vi "Serial_Auslesen_CO2Konzentration.vi"() -> ()   [LabVIEW 2023]
uses:
  aadfed2e-1559-dc4c-aa5c-28296088e4ea.vi
  <vilib>/Utility/file.llb/Write Delimited Spreadsheet (DBL).vi
  <vilib>/ptbypt/NI_PtbyPt.lvlib
panel:
  out "Mean CO2 Konzentration":dbl(graph)
  in  "Ref CO2":bool
  in  "Transmission Ref*1000:":i32
  in  "Verstärkung CO2:":i32
  in  "Verstärkung Ref:":i32
  out "CO2 Konzentration":dbl(graph)
  in  "Faktor Ch(CO2)*1000:":i32
  in  "Faktor CH(Referenz)*1000:":i32
  in  "Faktor k*1000:":i32
  in  "Abstand in cm:":i32
  in  "Absorbtionskoeffizient(CO2)*1000:":i32
  out "Mean Ref":dbl(graph)
  in  "Boolean":bool caption="In V aufnehmen"
  out "Mean A[V]:":dbl
  out "Aufnahme":dbl[](graph)
  in  "Aufnahme":bool
  in  "File":path
  in  "Transmit":bool
  in  "Sensor:":i8(knob) scale=1.0..4.0
  out "akt. Amplitude[V]:":dbl
  out "Mean Sig":dbl(graph)
  out "Ref":dbl(graph)
  in  "?":bool
  out "Waveform Chart":dbl(graph)
  in  "IR-Platine:":refnum<visa-resource-name>
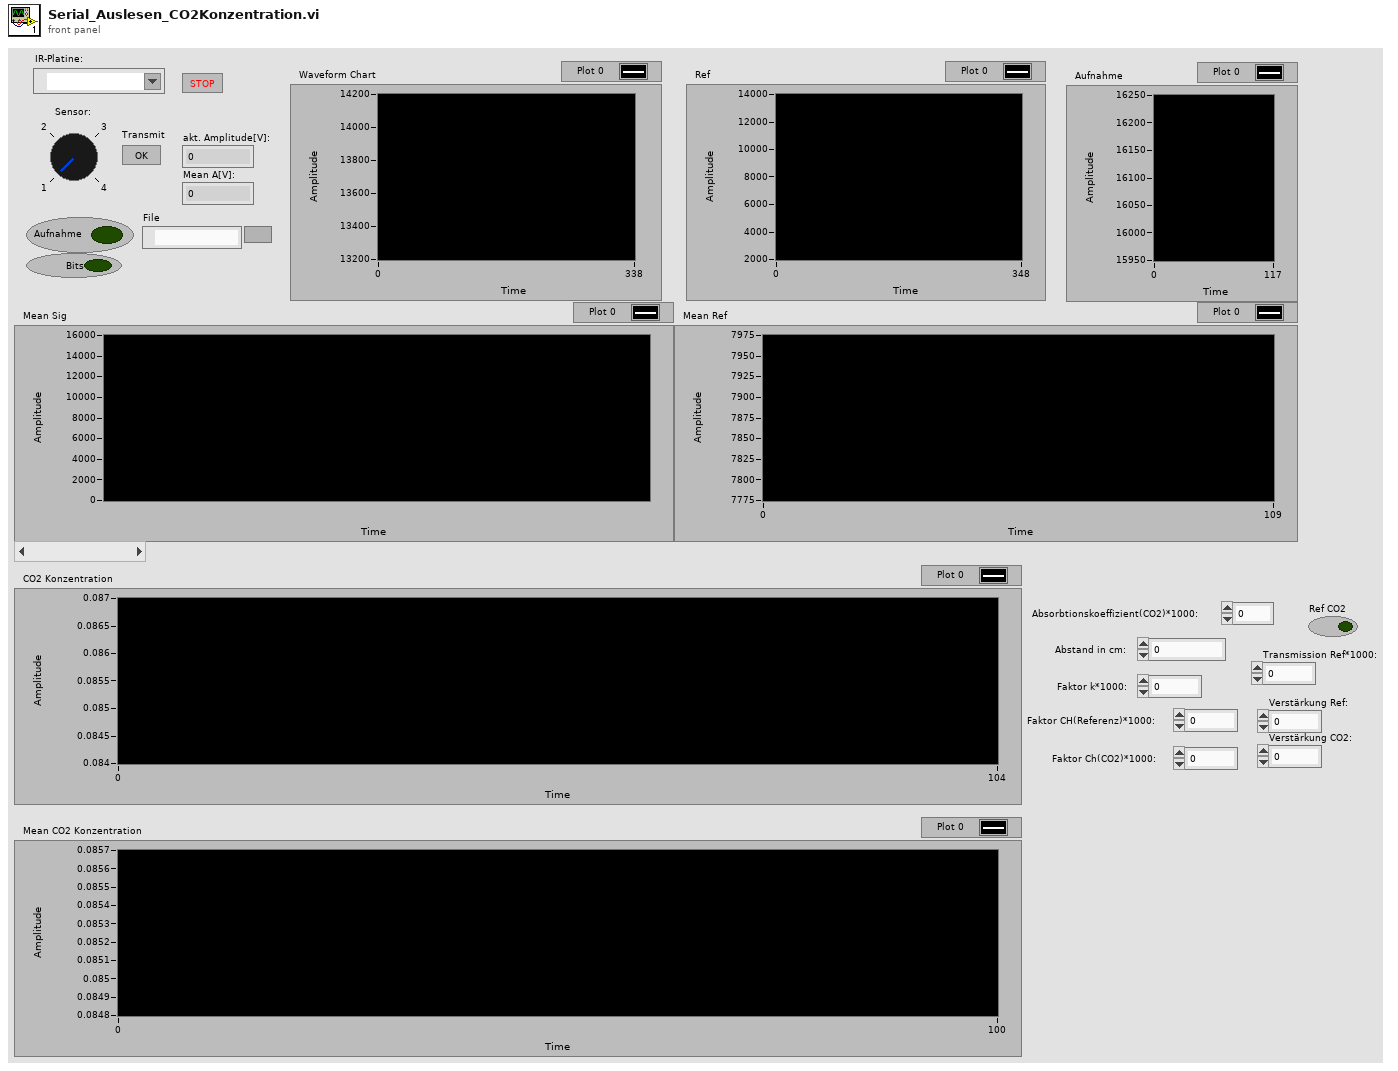
[diagram p1: front panel]
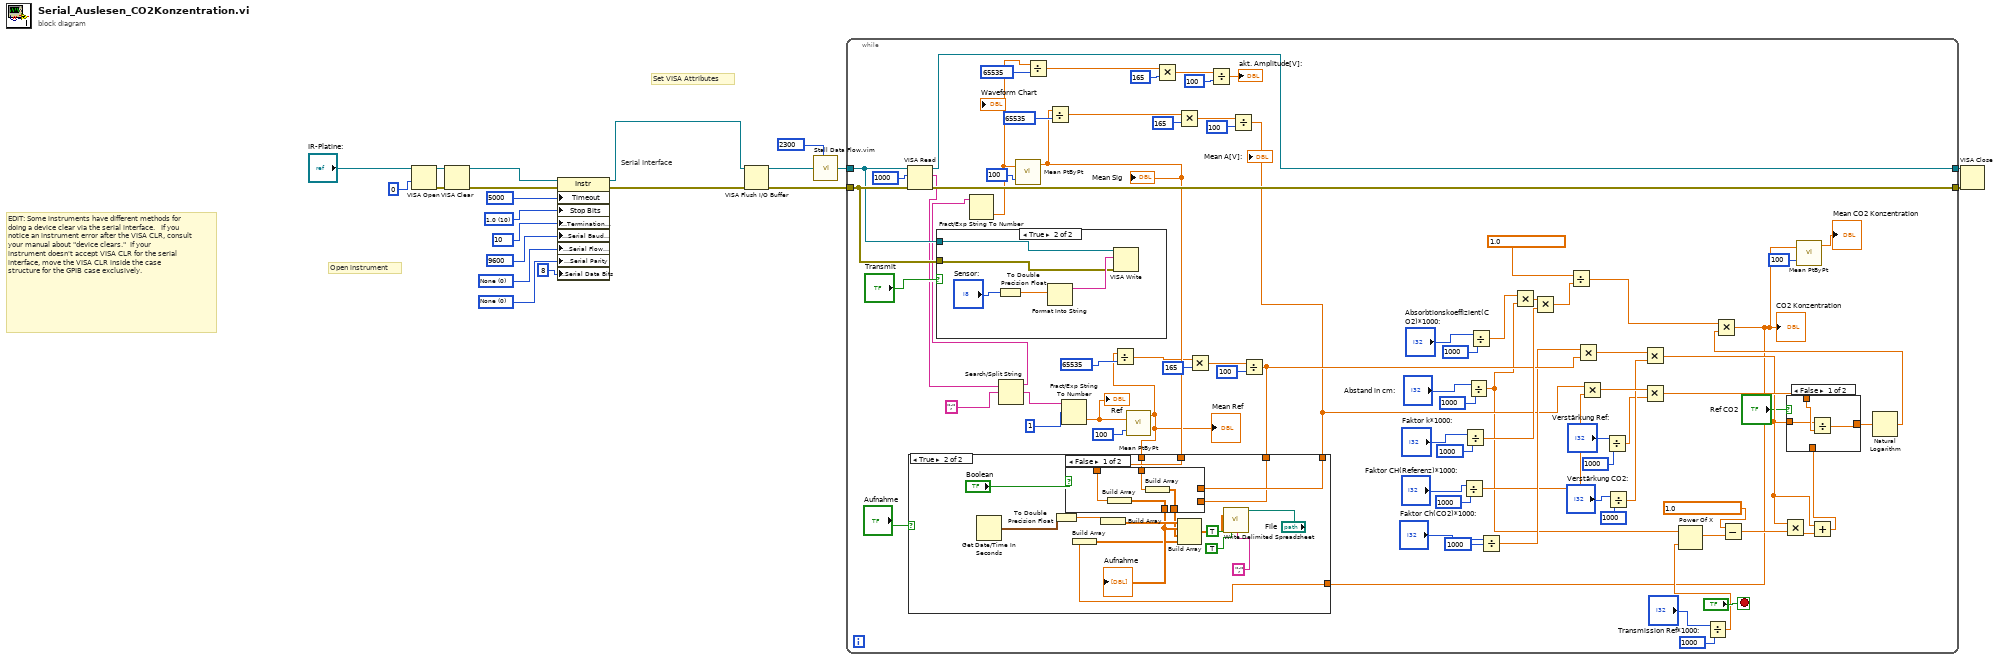
[diagram p0: block diagram]
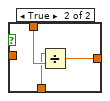
[diagram p2: hidden frame]
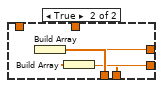
[diagram p4: hidden frame]
diagram:
  w9 = u16 0 items=["None", "Odd", "Even", "Mark", "Space"] ("Serial Settings:Parity")
  w10 = u16 0 items=["None", "XON/XOFF", "RTS/CTS", "XON/XOFF & RTS/CTS", "DTR/DSR", "XON/XOFF & DTR/DSR"] ("Serial Settings:Flow Control")
  w13 = u16 10 items=["1.0"=10, "1.5"=15, "2.0"=20] ("Serial Settings:Stop Bits")
  # "Serial Interface"
  # "EDIT: Some instruments have different methods for doing a device clear via the serial interface.   If you notice an instrument error after the VISA CLR, consult your manual about \"device clears.\"  If your instrument doesn't accept VISA CLR for the serial interface, move the VISA CLR inside the case  structure for the GPIB case exclusively."
  # "Set VISA Attributes"
  # "Open instrument"
  n1 = VISA Open(access mode=u32 0, VISA resource name="IR-Platine:") -> (VISA resource name=w19:refnum<visa-resource-name>, error out=w18:errorcluster)  [unwired: 3 in]
  n2 = VISA Clear(VISA resource name=w19, error in (no error)=w18) -> (VISA resource name out=w15:refnum<visa-resource-name>, error out=w1:errorcluster)
  n3 = property class="Instr"(reference=w15, error in=w1, "Timeout"=u32 5000 ("General Settings:Timeout Value"), "Stop Bits"=w13, "Message Based Settings:Termination Character"=u8 10, "Serial Settings:Serial Baud Rate"=u32 9600 ("Serial Settings:Baud Rate"), "Serial Settings:Serial Flow Control"=w10, "Serial Settings:Serial Parity"=w9, "Serial Settings:Serial Data Bits"=u16 8 ("Serial Settings:Data Bits")) -> (reference out=w16:refnum<visa-resource-name>, error out=w17:errorcluster)
  n4 = VISA Flush I/O Buffer(VISA resource name=w16, error in (no error)=w17) -> (VISA resource name out=w2:refnum<visa-resource-name>, error out=w3:errorcluster)  [unwired: 1 in]
  n5 = call "Stall Data Flow.vim"("value in"=w2, "milliseconds to wait"=u32 2300) -> ("value out"=w6:refnum<visa-resource-name>)  [unwired: 1 out]
  n6 = while {
    tunnel: w6 -> [w89]
    tunnel: w3 -> [w90]
    tunnel: [w99] -> w5
    tunnel: [w98] -> w4
    stop <- "?" stop-if-true
    n7 = VISA Read(VISA resource name=w89, byte count=u32 1000, error in (no error)=w90) -> (VISA resource name out=w99:refnum<visa-resource-name>, read buffer=w79:string, error out=w98:errorcluster)  [unwired: 1 out]
    n8 = case shown="True" "Transmit" {
      tunnel: w90 -> [_ w134]
      tunnel: w89 -> [_ w133]
      frame False {
      }
      frame True {
        n9 = To Double Precision Float(number="Sensor:") -> (double precision float=w136:dbl)
        n10 = Format Into String(w136) -> (resulting string=w135:string)  [unwired: 3 in, 1 out]
        n11 = VISA Write(VISA resource name=w133, write buffer=w135, error in (no error)=w134) -> ()  [unwired: 3 out]
      }
    }
    n12 = Search/Split String(string=w79, search string/char (-)=";") -> (substring before match=w78:string, match + rest of string=w76:string)  [unwired: 1 in, 1 out]
    n13 = Fract/Exp String To Number(string=w78) -> (number=w81:dbl)  [unwired: 3 in, 1 out]
    "Waveform Chart" <- w81
    n14 = call <vilib>:"Mean PtByPt.vi"("x"=w81, "sample length"=100) -> ("mean"=w80:dbl)  [unwired: 2 in, 1 out]
    "Mean Sig" <- w80
    n15 = Divide(x=w81, y=65535) -> (x/y=w95:dbl)
    n16 = Divide(x=w80, y=65535) -> (x/y=w83:dbl)
    n17 = Fract/Exp String To Number(string=w76, offset=1) -> (number=w68:dbl)  [unwired: 2 in, 1 out]
    "Ref" <- w68
    n18 = call <vilib>:"Mean PtByPt.vi"("x"=w68, "sample length"=100) -> ("mean"=w69:dbl)  [unwired: 2 in, 1 out]
    "Mean Ref" <- w69
    n19 = Divide(x=w69, y=65535) -> (x/y=w71:dbl)
    n20 = Multiply(x=w95, y=165) -> (x*y=w94:dbl)
    n21 = Multiply(x=w83, y=165) -> (x*y=w85:dbl)
    n22 = Multiply(x=w71, y=165) -> (x*y=w73:dbl)
    n23 = Divide(x=w94, y=100) -> (x/y=→"akt. Amplitude[V]:":dbl)
    n24 = Divide(x=w85, y=100) -> (x/y=w50:dbl)
    "Mean A[V]:" <- w50
    n25 = Divide(x=w73, y=100) -> (x/y=w52:dbl)
    n26 = Divide(x="Faktor CH(Referenz)*1000:", y=1000) -> (x/y=w49:dbl)
    n27 = Divide(x="Faktor k*1000:", y=1000) -> (x/y=w55:dbl)
    n28 = Divide(x="Abstand in cm:", y=1000) -> (x/y=w29:dbl)
    n29 = Divide(x="Absorbtionskoeffizient(CO2)*1000:", y=1000) -> (x/y=w56:dbl)
    n30 = Divide(x="Faktor Ch(CO2)*1000:", y=1000) -> (x/y=w51:dbl)
    n31 = Multiply(x=w56, y=w29) -> (x*y=w65:dbl)
    n32 = Multiply(x=w65, y=w55) -> (x*y=w54:dbl)
    n33 = Divide(x=1.0, y=w54) -> (x/y=w53:dbl)
    n34 = Multiply(x=w51, y=w52) -> (x*y=w46:dbl)
    n35 = Multiply(x=w50, y=w49) -> (x*y=w47:dbl)
    n36 = Divide(x="Verstärkung Ref:", y=1000) -> (x/y=w23:dbl)
    n37 = Divide(x="Verstärkung CO2:", y=1000) -> (x/y=w26:dbl)
    n38 = Multiply(x=w46, y=w26) -> (x*y=w35:dbl)
    n39 = Multiply(x=w47, y=w23) -> (x*y=w38:dbl)
    n40 = Divide(x="Transmission Ref*1000:", y=1000) -> (x/y=w39:dbl)
    n41 = Power Of X(1:w39, 2:w29) -> (0:w44:dbl)
    n42 = Subtract(x=1.0, y=w44) -> (x-y=w43:dbl)
    n43 = Multiply(x=w35, y=w43) -> (x*y=w42:dbl)
    n44 = Add(x=w35, y=w42) -> (x+y=w37:dbl)
    n45 = case shown="False" "Ref CO2" {
      tunnel: w38 -> [w103 w107]
      tunnel: w37 -> [_ w106]
      tunnel: [w104 w105] -> w36
      tunnel: w35 -> [w102 _]
      frame False {
        n46 = Divide(x=w102, y=w103) -> (x/y=w104:dbl)
      }
      frame True {
        n47 = Divide(x=w106, y=w107) -> (x/y=w105:dbl)
      }
    }
    n48 = Natural Logarithm(1:w36) -> (0:w48:dbl)
    n49 = Multiply(x=w53, y=w48) -> (x*y=w33:dbl)
    "CO2 Konzentration" <- w33
    n50 = case shown="True" "Aufnahme" {
      tunnel: w50 -> [_ w117]
      tunnel: w80 -> [_ w116]
      tunnel: w69 -> [_ w112]
      tunnel: w52 -> [_ w110]
      tunnel: w33 -> [_ w109]
      frame False {
      }
      frame True {
        n51 = Get Date/Time In Seconds() -> (seconds since 1Jan1904=w113:timestamp)
        n52 = To Double Precision Float(number=w113) -> (double precision float=w114:dbl)
        n53 = case shown="False" "Boolean" {
          tunnel: w117 -> [_ w131]
          tunnel: w116 -> [w128 _]
          tunnel: [w127 w132] -> w115
          tunnel: w112 -> [w126 _]
          tunnel: [w125 w129] -> w111
          tunnel: w110 -> [_ w130]
          frame False {
            n54 = Build Array(w128) -> (w127:dbl[])
            n55 = Build Array(w126) -> (w125:dbl[])
          }
          frame True {
            n56 = Build Array(w131) -> (w132:dbl[])
            n57 = Build Array(w130) -> (w129:dbl[])
          }
        }
        "Aufnahme" <- w115
        n58 = Build Array(w109) -> (w108:dbl[])
        n59 = Build Array(w114) -> (w119:dbl[])
        n60 = Build Array(w119, w115, w111, w108) -> (w120:dbl[][])
        n61 = call-poly <vilib>:"Write Delimited Spreadsheet.vi"("file path (dialog if empty)"="File", "2D data"=w120, "append to file? (new file:F)"=TRUE, "transpose? (no:F)"=TRUE, "delimiter (\\t)"=";" ("delimiter (\\t)")) -> ()  [unwired: 9 in, 2 out]
      }
    }
    n62 = call <vilib>:"Mean PtByPt.vi"("x"=w33, "sample length"=100) -> ("mean"=→"Mean CO2 Konzentration":dbl)  [unwired: 2 in, 1 out]
  }
  n63 = VISA Close(VISA resource name=w5, error in (no error)=w4) -> ()  [unwired: 1 out]
